vi "LED-Change text.vi"(5 "Container State":T1, 6 "LED Display":refnum<vi>, 7 "vi reference in":refnum<vi>, 8 "Should Change?":bool, 9 "Data In":T2) -> (1 "vi reference out":refnum<vi>, 3 "Data Out":T2)   [LabVIEW 2011, in "LED Display.xctl"]
uses:
  LED Display.xctl
  LED-Data.ctl
  <vilib>/_xctls/Container State.ctl
  <vilib>/_xctls/XControlSupport.lvlib
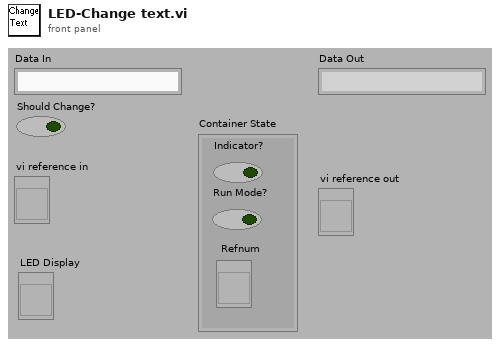
[diagram p1: front panel]
types:
  T1 = typedef "XControlSupport.lvlib/Container State.ctl" = cluster{"Indicator?":bool, "Run Mode?":bool, " Refnum":refnum<vi>}
  T2 = typedef "LED Display.xctl/LED-Data.ctl" = string
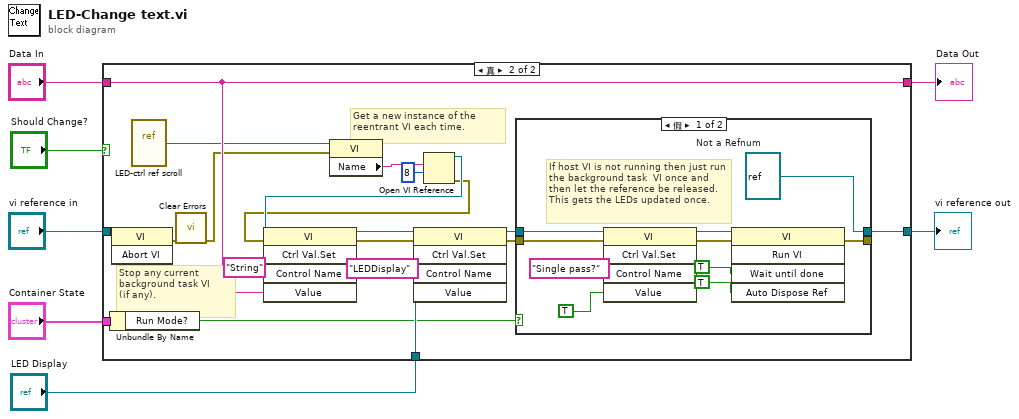
[diagram p0: block diagram]
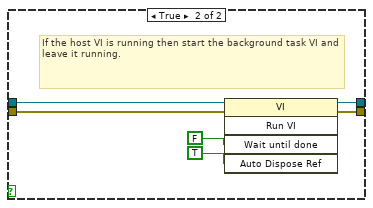
[diagram p3: hidden frame]
diagram:
  n1 = case shown="真" "Should Change?" {
    tunnel: "Data In" -> [w8 w25]
    tunnel: "vi reference in" -> [w9 w28]
    tunnel: [w9 w27] -> w4
    tunnel: "Container State" -> [_ w26]
    tunnel: [w8 w25] -> w3
    tunnel: "LED Display" -> [_ w24]
    frame False {
    }
    frame True {
      # "Stop any current\nbackground task VI\n(if any)."
      # "Get a new instance of the \nreentrant VI each time."
      n2 = Unbundle By Name(w26) -> ("Run Mode?"=w23:bool)
      n3 = invoke class="VI" method="Abort VI"(reference=w28) -> (error out=w10:errorcluster)  [unwired: 2 in, 2 out]
      n4 = vi-ref "LED-ctrl ref scroll.vi"() -> (w18:refnum<vi>)
      n5 = call <vilib>:"Clear Errors.vi"("error in (no error)"=w10) -> ("error out"=w11:errorcluster)  [unwired: 6 in]
      n6 = property class="VI"(reference=w18, error in=w11) -> ("Name"=w17:string)  [unwired: 2 out]
      n7 = Open VI Reference(vi path=w17, options=8) -> (vi reference=w16:refnum<vi>, error out=w12:errorcluster)  [unwired: 4 in]
      n8 = invoke class="VI" method="Ctrl Val.Set"(reference=w16, error in=w12, "Control Name"="String", "Value"=w25) -> (reference out=w21:refnum<vi>, error out=w20:errorcluster)  [unwired: 1 in, 3 out]
      n9 = invoke class="VI" method="Ctrl Val.Set"(reference=w21, error in=w20, "Control Name"="LEDDisplay", "Value"=w24) -> (reference out=w14:refnum<vi>, error out=w13:errorcluster)  [unwired: 1 in, 3 out]
      n10 = case shown="假" w23 {
        tunnel: [w38 w42] -> w27
        tunnel: w14 -> [w34 w41]
        tunnel: w13 -> [w31 w40]
        tunnel: [w29 w39] -> _
        frame False {
          w38 = refnum<vi> refnum  # Not a Refnum
          # "If host VI is not running then just run the background task  VI once and then let the reference be released. This gets the LEDs updated once."
          n11 = invoke class="VI" method="Ctrl Val.Set"(reference=w34, error in=w31, "Control Name"="Single pass?", "Value"=TRUE ("Auto Dispose Reference")) -> (reference out=w33:refnum<vi>, error out=w32:errorcluster)  [unwired: 1 in, 3 out]
          n12 = invoke class="VI" method="Run VI"(reference=w33, error in=w32, "Wait until done"=TRUE ("Wait Until Done"), "Auto Dispose Ref"=TRUE ("Auto Dispose Reference")) -> (error out=w29:errorcluster)  [unwired: 1 in, 4 out]
        }
        frame True {
          # "If the host VI is running then start the background task VI and leave it running."
          n13 = invoke class="VI" method="Run VI"(reference=w41, error in=w40, "Wait until done"=FALSE ("Wait Until Done"), "Auto Dispose Ref"=TRUE ("Auto Dispose Reference")) -> (reference out=w42:refnum<vi>, error out=w39:errorcluster)  [unwired: 1 in, 3 out]
        }
      }
    }
  }
  "vi reference out" <- w4
  "Data Out" <- w3
